vi "Redraw Event FGV.vi"(8 "error in (no error)":errorcluster, 11 "Action (Get)":enum16{"Get", "Destroy"}(ring)) -> (0 "error out":errorcluster, 3 "Redraw Event":refnum<user-event>)   [LabVIEW 2019, in "SLSC Switch System Explorer.lvlib"]
uses:
  SLSC Switch System Explorer.lvlib
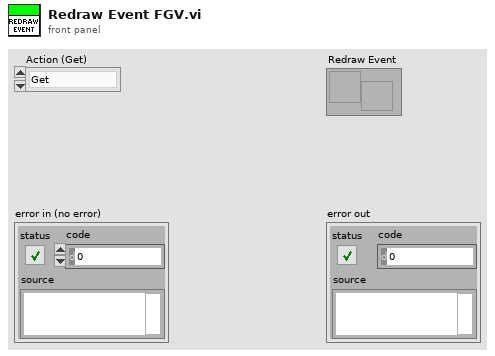
[diagram p1: front panel]
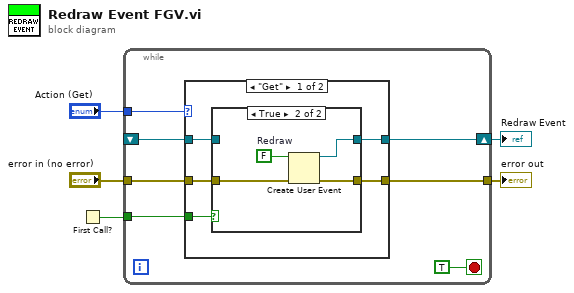
[diagram p0: block diagram]
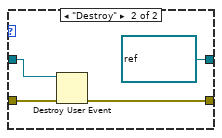
[diagram p3: hidden frame]
diagram:
  n1 = First Call?() -> (First Call?: T/F=w5:bool)
  n2 = while {
    tunnel: w5 -> [w12]
    tunnel: "error in (no error)" -> [w11]
    tunnel: "Action (Get)" -> [w10]
    tunnel: [w9] -> w2
    shift-right: [w8] -> w1
    shift-left: _ -> [w6]
    stop <- TRUE stop-if-true
    n3 = case shown="\"Get\"" w10 {
      tunnel: w12 -> [w17 _]
      tunnel: w11 -> [w16 w27]
      tunnel: [w15 w24] -> w9
      tunnel: [w14 refnum<user-event> refnum ("Redraw")] -> w8
      tunnel: w6 -> [w13 w26]
      frame "Get" {
        n4 = case shown="True" w17 {
          tunnel: w16 -> [w19 w22]
          tunnel: [w19 w21] -> w15
          tunnel: [w18 w20] -> w14
          tunnel: w13 -> [w18 _]
          frame False {
          }
          frame True {
            w23 = FALSE  # Redraw
            n5 = Create User Event(user event datatype=w23, error in=w22) -> (user event=w20:refnum<user-event>, error out=w21:errorcluster)
          }
        }
      }
      frame "Destroy" {
        n6 = Destroy User Event(user event=w26, error in=w27) -> (error out=w24:errorcluster)
      }
    }
  }
  "error out" <- w2
  "Redraw Event" <- w1
